vi "Init DC meter.vi"(8 "error in (no error)":errorcluster, 11 "DC meter":T1={"DC meter type"=enum."H/A/K 3458", "DC meter VISA"="", "NPLC"=10.0, "status ref"=refnum}) -> (0 "error out":errorcluster, 2 "Init status":string, 3 "DC meter out":T1={"DC meter type"=enum."H/A/K 3458", "DC meter VISA"="", "NPLC"=10.0, "status ref"=refnum})   [LabVIEW 2020]
doc: "Initialize the driver of the selected DC meter."
uses:
  Type definitions/DC meter.ctl
  Type definitions/DC meter type.ctl
  external libraries/Fluke 8508/Fluke 8508.lvlib
  external libraries/3458A Basic Driver/3458A Basic Driver.lvlib
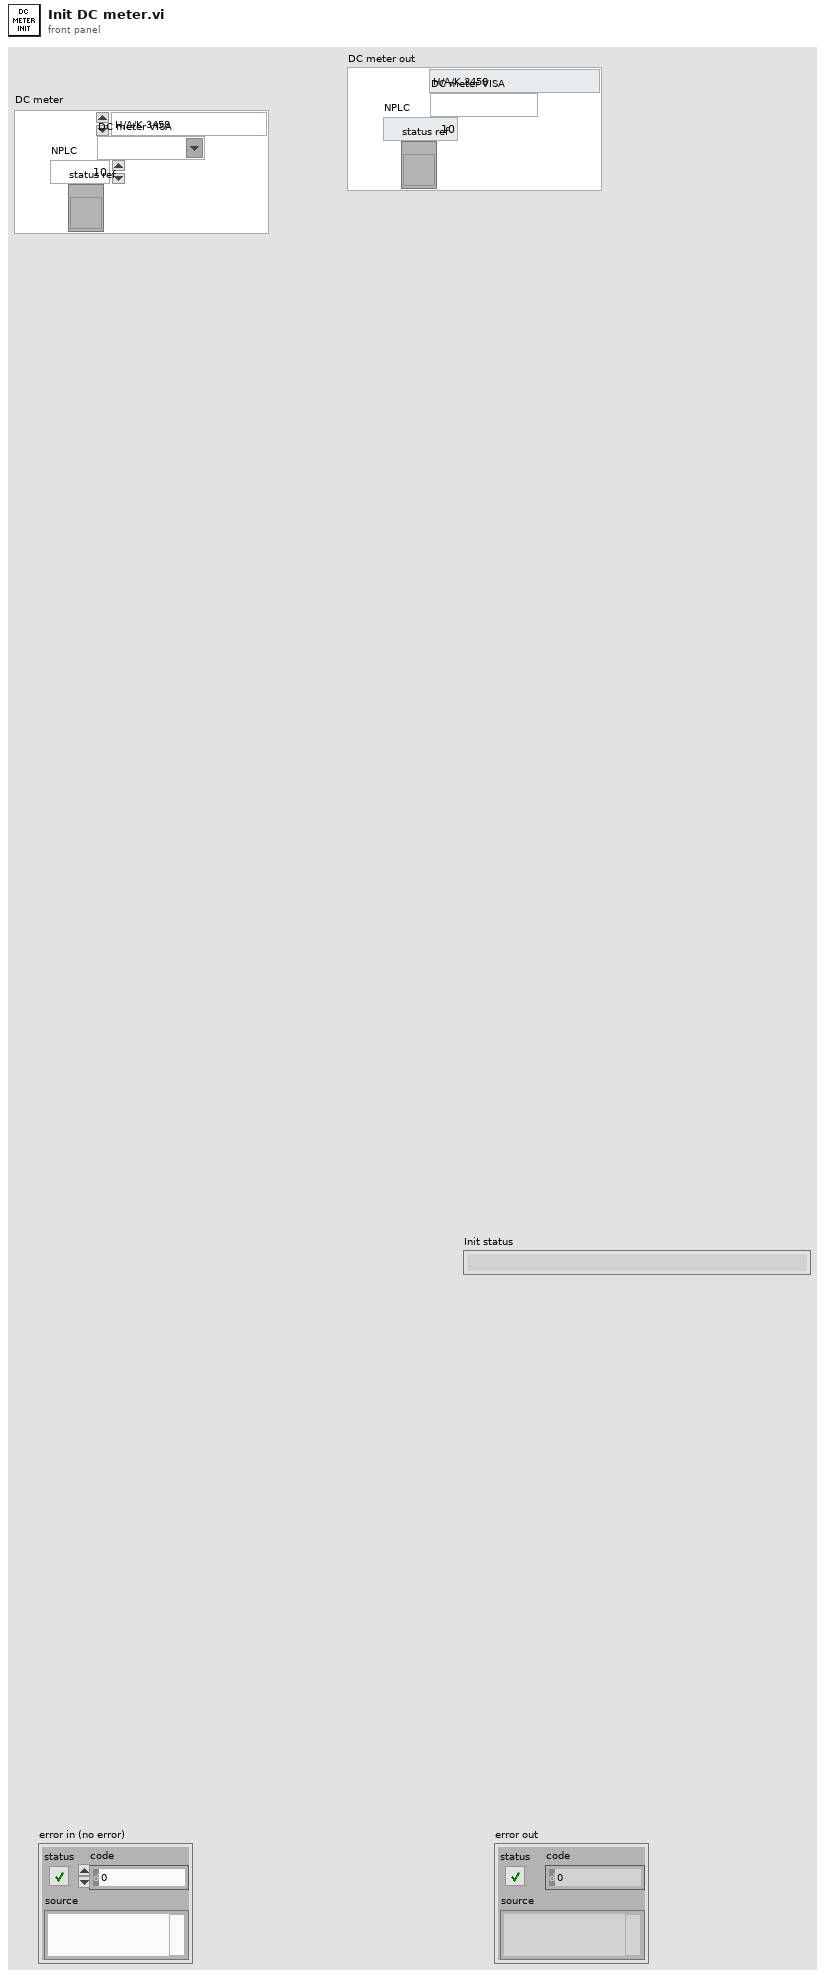
[diagram p1: front panel]
types:
  T1 = typedef "DC meter.ctl" = cluster{"DC meter type":T2, "DC meter VISA":refnum<visa-resource-name>, "NPLC":dbl, "status ref":refnum<vi>}
  T2 = typedef "DC meter type.ctl" = enum16{"H/A/K 3458", "Fluke 8508A", "dummy", "Keithley 2182"}
  T3 = cluster{"error":bool, "code":i32, "source":string}
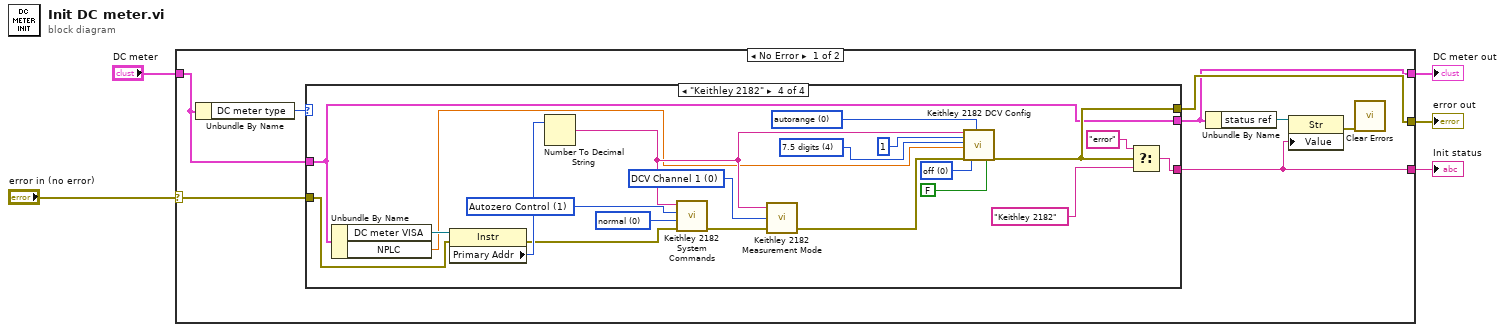
[diagram p0: block diagram]
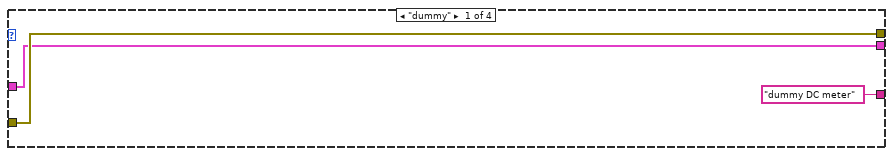
[diagram p2: hidden frame]
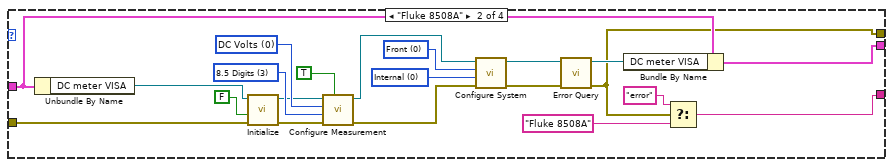
[diagram p3: hidden frame]
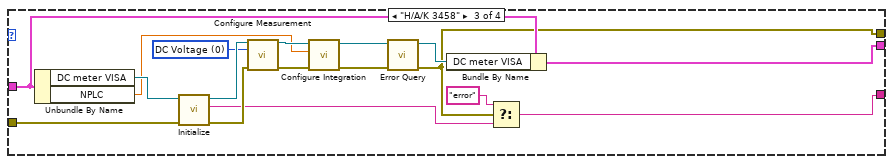
[diagram p4: hidden frame]
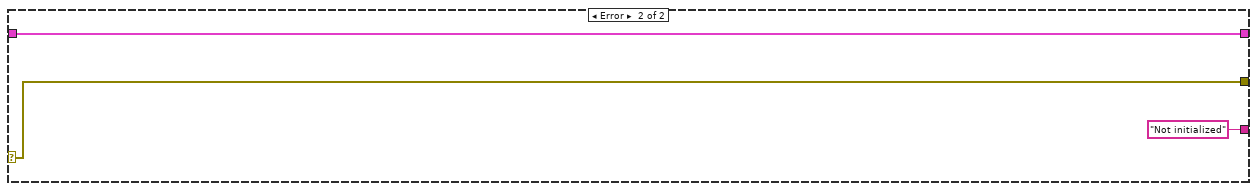
[diagram p5: hidden frame]
diagram:
  n1 = case shown="No Error" "error in (no error)" {
    selector: "error in (no error)" -> [w10 w78]
    tunnel: [w13 w78] -> w5
    tunnel: [w7 "Not initialized" ("idn string")] -> w4
    tunnel: "DC meter" -> [w11 w77]
    tunnel: [w9 w77] -> w2
    frame No Error {
      n2 = Unbundle By Name(w11) -> ("DC meter type"=w12:T2)
      n3 = case shown="\"Keithley 2182\"" w12 {
        tunnel: w10 -> [w16 w36 w54 w61]
        tunnel: [w16 w18 w41 w57] -> w13
        tunnel: w11 -> [w15 w25 w50 w55]
        tunnel: [w15 w24 w49 w55] -> w9
        tunnel: ["dummy DC meter" ("idn string") w17 w39 w56] -> w7
        frame "dummy" {
        }
        frame "Fluke 8508A" {
          w26 = u16 0 items=["Internal", "External"] ("Guard (0: Internal)")
          w27 = u16 0 items=["Front", "Rear", "Ratio", "Difference", "Deviation", "OFF"] ("Terminals (0: Front)")
          w33 = 3 items=["5.5 Digits", "6.5 Digits", "7.5 Digits", "8.5 Digits"] ("Resolution (1: 6.5 Digits)")
          w34 = u16 0 items=["DC Volts", "AC Volts", "DC Current", "AC Current", "Normal Resistance", "High Voltage Resistance", "True Resistance"] ("Function (0: DC Volts)")
          n4 = Unbundle By Name(w25) -> ("DC meter VISA"=w37:refnum<visa-resource-name>)
          n5 = call "Initialize.vi"("error in (no error)"=w36, "Reset? (T: Yes)"=FALSE, "VISA resource name"=w37) -> ("error out"=w31:errorcluster, "VISA resource name out"=w32:refnum<visa-resource-name>)  [unwired: 7 in]
          n6 = call "Configure Measurement.vi"("Enable Auto Range (True)"=TRUE, "error in (no error)"=w31, "Resolution (1: 6.5 Digits)"=w33, "Function (0: DC Volts)"=w34, "VISA resource name"=w32) -> ("error out"=w29:errorcluster, "VISA resource name out"=w30:refnum<visa-resource-name>)  [unwired: 5 in]
          n7 = call "Configure System.vi"("error in (no error)"=w29, "Guard (0: Internal)"=w26, "Terminals (0: Front)"=w27, "VISA resource name"=w30) -> ("error out"=w23:errorcluster, "VISA resource name out"=w22:refnum<visa-resource-name>)  [unwired: 6 in]
          n8 = call "Error Query.vi"("error in (no error)"=w23, "VISA resource name"=w22) -> ("error out"=w18:errorcluster, "VISA resource name out"=w21:refnum<visa-resource-name>)  [unwired: 6 in, 2 out]
          n9 = Bundle By Name(cluster=w25, "DC meter VISA"=w21) -> (w24:T1)
          n10 = Select(t="error" ("idn string"), s=w18, f="Fluke 8508A" ("idn string")) -> (s? t:f=w17:string)
        }
        frame "H/A/K 3458" {
          w42 = u16 0 items=["DC Voltage", "AC Voltage", "AC + DC Voltage", "DC Current", "AC Current", "AC + DC Current", "2-Wire Resistance", "4-Wire Resistance", "Frequency", "Period", "Direct Sampling DC", "Direct Sampling AC", "Sub-Sampling DC", "Sub-Sampling AC"] ("Function (0: DC Voltage)")
          n11 = Unbundle By Name(w50) -> ("DC meter VISA"=w48:refnum<visa-resource-name>, "NPLC"=w43:dbl)
          n12 = call "Initialize.vi"("error in (no error)"=w54, "VISA resource name"=w48) -> ("error out"=w53:errorcluster, "idn string"=w38:string, "VISA resource name out"=w47:refnum<visa-resource-name>)  [unwired: 7 in]
          n13 = call "Configure Measurement.vi"("VISA resource name"=w47, "Function (0: DC Voltage)"=w42, "error in (no error)"=w53) -> ("VISA resource name out"=w46:refnum<visa-resource-name>, "error out"=w52:errorcluster)  [unwired: 11 in]
          n14 = call "Configure Integration.vi"("error in (no error)"=w52, "Integration Time (0 PLCs)"=w43, "VISA resource name"=w46) -> ("error out"=w51:errorcluster, "VISA resource name out"=w45:refnum<visa-resource-name>)  [unwired: 7 in]
          n15 = call "Error Query.vi"("error in (no error)"=w51, "VISA resource name"=w45) -> ("error out"=w41:errorcluster, "VISA resource name out"=w44:refnum<visa-resource-name>)  [unwired: 6 in, 2 out]
          n16 = Bundle By Name(cluster=w50, "DC meter VISA"=w44) -> (w49:T1)
          n17 = Select(t="error" ("idn string"), s=w41, f=w38) -> (s? t:f=w39:string)
        }
        frame "Keithley 2182" {
          w65 = u16 0 items=["off", "moving filter", "repeating filter"] ("digital filter (off:0)")
          w67 = u16 4 items=["3.5 digits", "4.5 digits", "5.5 digits", "6.5 digits", "7.5 digits"] ("resolution (6.5 digits:3)")
          w69 = u16 0 items=["autorange", "set range value"] ("range (auto:0)")
          w70 = u16 0 items=["DCV Channel 1", "DCV Channel 2", "Temperature Channel 1", "Temperature Channel 2", "Ratio Mode On", "Ratio Mode Off", "Delta Mode On", "Delta Mode Off", "Internal Temperature Sensor"] ("Measurement Mode Select")
          w74 = u16 0 items=["normal", "disable"] ("autozero (normal:0)")
          w75 = u16 1 items=["Return to System Preset Defaults", "Autozero Control", "Line Cycle Synchronization", "Select Power-On Setup", "Save Setup SAV0", "Recall Saved Setup SAV0", "Clear Error Message Queue", "Key Click Control", "Limit Beeper Control", "Simulate Key Press"] ("System Command Functions")
          n18 = Unbundle By Name(w55) -> ("DC meter VISA"=w73:refnum<visa-resource-name>, "NPLC"=w66:dbl)
          n19 = property class="Instr"(reference=w73, error in=w61) -> (error out=w60:errorcluster, "Primary Addr"=w72:u16)  [unwired: 1 out]
          n20 = Number To Decimal String(number=w72) -> (decimal integer string=w71:string)  [unwired: 1 in]
          n21 = call "Keithley 2182 System Commands.vi"("error in"=w60, "autozero (normal:0)"=w74, "System Command Functions"=w75, "GPIB address"=w71) -> ("error out"=w62:T3)  [unwired: 7 in]
          n22 = call "Keithley 2182 Measurement Mode.vi"("error in"=w62, "Measurement Mode Select"=w70, "GPIB Address"=w71) -> ("error out"=w63:T3)  [unwired: 2 in]
          n23 = call "Keithley 2182 DCV Config.vi"("GPIB address"=w71, "Channel to Configure"=i8 1, "resolution (6.5 digits:3)"=w67, "Number Power Line Cycles"=w66, "error in"=w63, "digital filter (off:0)"=w65, "range (auto:0)"=w69, "Low Pass Analog Filter Control"=FALSE) -> ("error out"=w57:T3)  [unwired: 11 in]
          n24 = Select(t="error" ("idn string"), s=w57, f="Keithley 2182" ("idn string")) -> (s? t:f=w56:string)
        }
      }
      n25 = Unbundle By Name(w9) -> ("status ref"=w8:refnum<vi>)
      n26 = property class="Str"(reference=w8, "Value"=w7) -> (error out=w6:errorcluster)  [unwired: 1 in, 1 out]
      n27 = call <vilib>:"Clear Errors.vi"("error in (no error)"=w6) -> ()  [unwired: 5 in, 2 out]
    }
    frame Error {
    }
  }
  "error out" <- w5
  "Init status" <- w4
  "DC meter out" <- w2
